vi "Test Format Method Execution Time.vi"(8 "error in (no error)":errorcluster, 11 "Test Result Tree Test in":refnum<class "Test Result Tree Test.lvclass">) -> (0 "error out":errorcluster, 3 "Test Result Tree Test out":refnum<class "Test Result Tree Test.lvclass">)   [LabVIEW 2020, in "Test Result Tree Test.lvclass"]
uses:
  Test Result Tree Test.lvclass
  C:/Program Files (x86)/National Instruments/LabVIEW 2020/vi.lib/Astemes/LUnit/Test Case.lvclass
  Test Result Tree/Test Result Tree V2.lvclass
  C:/Git/astemes-lunit/source/Rewrite Project/Test Tree/Test Tree.lvclass
  LUnit Test Case Tests/LUnit Test Case V2 Test Double/Methods.ctl
  <vilib>/Astemes/LUnit/Test Case.lvclass/Test Case.ctl
  3218c730-9013-45aa-9bf9-4d6791bb458c.vi
  <vilib>/Astemes/LUnit/Palette/Fail.vi
  <vilib>/Astemes/LUnit/Palette/Pass.vi
  <vilib>/Astemes/LUnit/Compare Variants.vi
  <vilib>/Astemes/LUnit/Describe Comparison.vi
  <vilib>/Astemes/LUnit/Set Assertion Type.vi
  <vilib>/Astemes/LUnit/Add test result.vi
  <vilib>/Astemes/LUnit/Variant to string.vi
  <vilib>/Astemes/LUnit/LUnit Record Assertion Result.vi
  <vilib>/Astemes/LUnit/LUnit Aggregate Assertion Results.vi
  <vilib>/Astemes/LUnit/Method Result/LUnit Merge Status.vi
  <vilib>/Astemes/LUnit/LUnit Concatenate result strings.vi
  <vilib>/Utility/Data Type/Get Type Information.vi
  <vilib>/Utility/LVClass/Get LV Class Name.vi
  LUnit Test Case/LUnit Test Case V2.lvclass
  Test Result Tree Test.lvclass/Test Result Tree Test.ctl
  Test Tree/Test Tree.lvclass
  LUnit Test Case Tests/LUnit Test Case V2 Test Double/LUnit Test Case V2 Test Double.lvclass
panel:
  out "Description":string
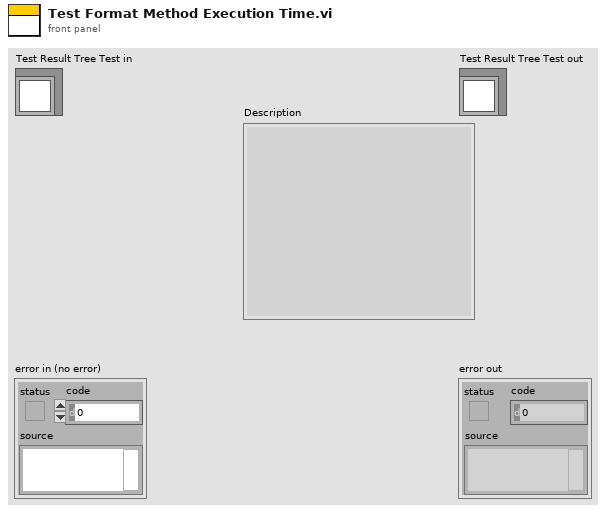
[diagram p1: front panel]
types:
  T1 = typedef "LUnit Test Case V2 Test Double.lvclass/Methods.ctl" = enum16{"Test Failing Test.vi", "Test Passing Test.vi", "Test Error Test.vi", "Test Skip Test.vi", "Test Passing Pass If Test.vi", "Test Failing Pass If Test.vi", "Test Failing Fail If Test.vi", "Test Passing Fail If Test.vi", "Test Passing Pass If Error Test.vi", "Test Failing Pass If Error Test.vi", "Test Passing Fail If Error Test.vi", "Test Failing Fail If Error Test.vi", "Test Passing Pass If Equal Test.vi", "Test Failing Pass If Equal Test.vi", "Test Failing Fail If Equal Test.vi", "Test Passing Fail If Equal Test.vi"}
  T2 = typedef "Result.lvlib/Result.ctl" = cluster{"Name":string, "Message":string, "Description":string, "Status":T3, "Result Type":T4, "Execution Time":dbl}
  T3 = typedef "Result.lvlib/Status.ctl" = enum16{"", "Passed", "Failed", "Error", "Skipped", "Setup Error", "Broken", "Teardown Error"}
  T4 = typedef "Result.lvlib/Type.ctl" = enum16{"Method", "Case", "Suite", "Pass", "Fail", "Skip", "Pass if", "Fail if", "Pass if Error", "Fail if Error", "Pass if Equal", "Fail if Equal"}
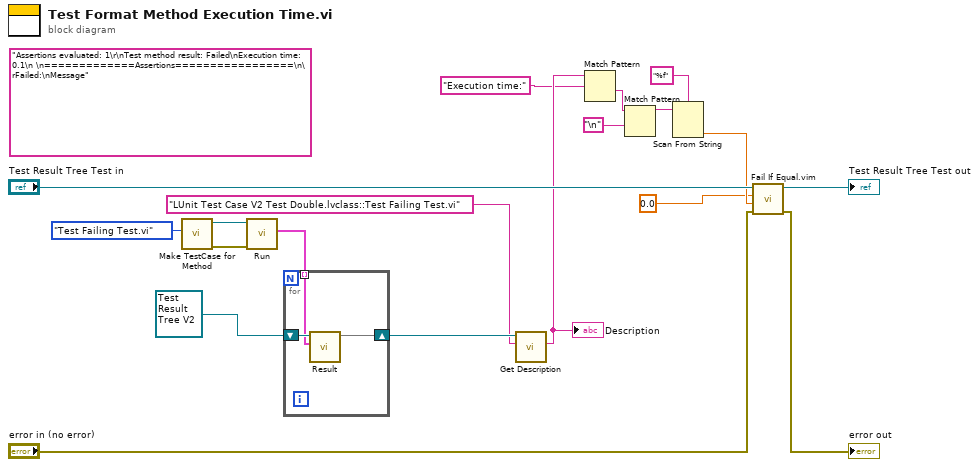
[diagram p0: block diagram]
diagram:
  (unwired) "Assertions evaluated: 1\r\nTest method result: Failed\nExecution time: 0.1\n \n=============Assertions=================\n\rFailed:\nMessage" ("format string")
  n1 = call "Make TestCase for Method.vi"("Test Method"=Methods."Test Failing Test.vi") -> ("error out"=w12:errorcluster, "LUnit Test Case V2 out"=w13:refnum<class "LUnit Test Case V2.lvclass">)  [unwired: 9 in]
  n2 = call-dynamic "Run.vi"("error in (no error)"=w12, "LUnit Test Case V2 in"=w13) -> ("Results"=w9:T2[])  [unwired: 8 in, 1 out]
  n3 = for {
    shift-right: [w22] -> w16
    shift-left: refnum<class "Test Result Tree V2.lvclass"> refnum ("Test Result Tree V2.lvclass") -> [w21]
    tunnel: w9 -> [w20] mode=indexing
    n4 = call-dynamic "Result.vi"("Result"=w20, "Test Result Tree V2 in"=w21) -> (3:w22)  [unwired: 8 in, 1 out]
  }
  n5 = call "Get Description.vi"("Tag"="LUnit Test Case V2 Test Double.lvclass::Test Failing Test.vi" ("Case"), "Test Tree In"=w16) -> ("Description"=w8:string)  [unwired: 6 in, 3 out]
  "Description" <- w8
  n6 = Match Pattern(string=w8, regular expression="Execution time:" ("format string")) -> (after substring=w6:string)  [unwired: 1 in, 3 out]
  n7 = Match Pattern(string=w6, regular expression="\n") -> (before substring=w4:string)  [unwired: 1 in, 3 out]
  n8 = Scan From String(format string="%f", input string=w4) -> (output 1=w2:dbl)  [unwired: 3 in, 3 out]
  n9 = call "Fail If Equal.vim"("error in (no error)"="error in (no error)", "Actual"=w2, "Expected"=0.0 ("output 1"), "LUnit Test Case In"="Test Result Tree Test in") -> ("error out"=→"error out":errorcluster, "LUnit Test Case Out"=→"Test Result Tree Test out":refnum<class "Test Result Tree Test.lvclass">)  [unwired: 6 in]
